vi "Shutdown.vi"(11 "Sequence Context In":refnum<k7>) -> (0 "error out":errorcluster)   [LabVIEW 2017]
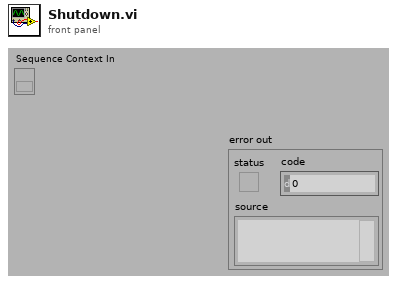
[diagram p1: front panel]
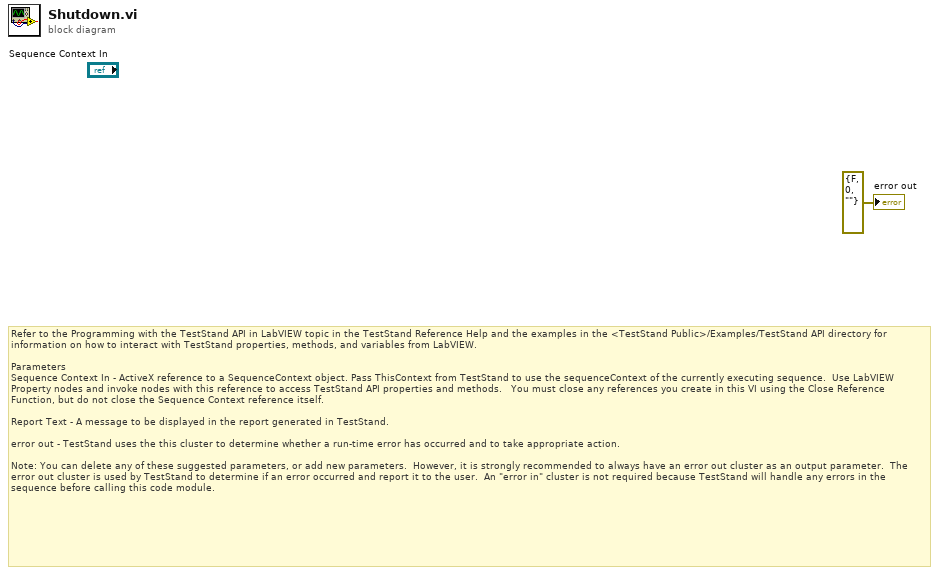
[diagram p0: block diagram]
diagram:
  # "Refer to the Programming with the TestStand API in LabVIEW topic in the TestStand Reference Help and the examples in the <TestStand Public>/Examples/TestStand API directory for information on how to interact with TestStand properties, methods, and variables from LabVIEW.\n\nParameters\nSequence Context In - ActiveX reference to a SequenceContext object. Pass ThisContext from TestStand to use the sequenceContext of the currently executing sequence.  Use LabVIEW Property nodes and invoke nodes with this reference to access TestStand API properties and methods.   You must close any references you create in this VI using the Close Reference Function, but do not close the Sequence Context reference itself.\n\nReport Text - A message to be displayed in the report generated in TestStand. \n\nerror out - TestStand uses the this cluster to determine whether a run-time error has occurred and to take appropriate action.  \n\nNote: You can delete any of these suggested parameters, or add new parameters.  However, it is strongly recommended to always have an error out cluster as an output parameter.  The error out cluster is used by TestStand to determine if an error occurred and report it to the user.  An \"error in\" cluster is not required because TestStand will handle any errors in the sequence before calling this code module."
  "error out" <- errorcluster {"status"=FALSE, "code"=0, "source"=""} ("error out")
